vi "Generate Window Title.vi"(10 "Module Name":string, 11 "Item Name":string) -> (3 "Window Title":string)   [LabVIEW 2020]
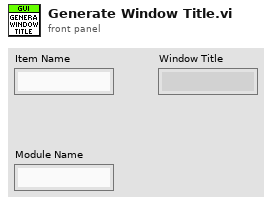
[diagram p1: front panel]
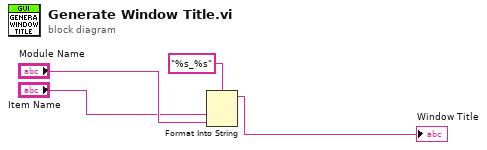
[diagram p0: block diagram]
diagram:
  n1 = Format Into String(format string="%s_%s", "Item Name", "Module Name") -> (resulting string=→"Window Title":string)  [unwired: 2 in, 1 out]
